vi "SP Format Marker Table.vi"(7 "CH Control In":T2={"Trace Orientation"=enum."Overlay", "Frequency"={"Change Frequency"=FALSE, "Start"=500.0, "Stop"=1500.0, "Units"=enum."MHz"}, "Markers"=[], "Traces"=[]} {"Traces"."Reference" format="%#.2g"; "Traces"."Display Data" items=["Data", "Memory", "Data/Memory"]; "Traces"."Format" items=["Log Mag", "Phase", "Expanded Phase", "Delay", "Smith", "Polar", "Lin Mag", "SWR", "Loss", "Real", "Imaginary"]; "Traces"."Scale" min=0.001 step=1.0 format="%#.2g"; "Traces"."Position" min=0.0 max=10.0; "Frequency"."Stop" format="%.3g"; "Frequency"."Start" format="%.3g"}, 8 "error in (no error)":errorcluster, 10 "Marker Table":refnum<vi>, 11 "Plot Ref":refnum<vi>) -> (0 "error out":errorcluster, 1 "Disable Button Values":T1)   [LabVIEW 2011]
uses:
  TypeDefs/SP Display Plot Controls Cluster.ctl
  TypeDefs/SP Frequency Units.ctl
  TypeDefs/SP Marker Cluster.ctl
  TypeDefs/SP Marker Type.ctl
  TypeDefs/SP Display Trace Controls.ctl
  TypeDefs/SP Display Format.ctl
  TypeDefs/SP Display Data.ctl
panel:
  # "Div"
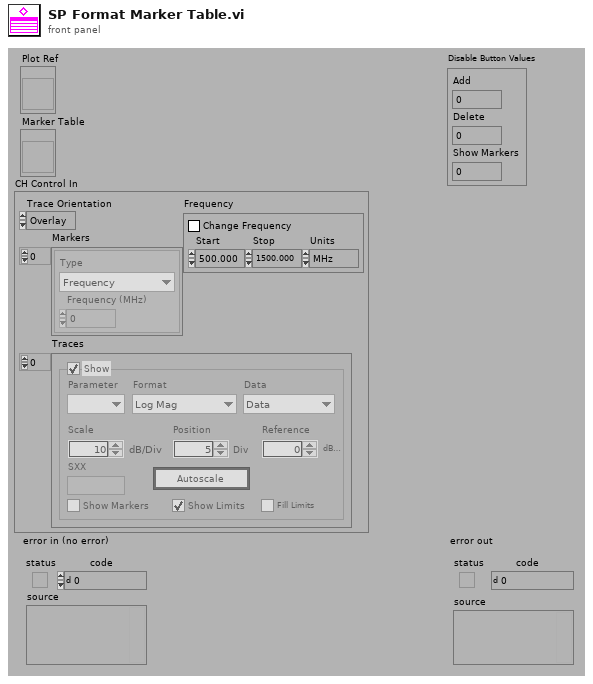
[diagram p1: front panel]
types:
  T1 = cluster{"Add":u8, "Delete":u8, "Show Markers":u8}
  T2 = typedef "SP Display Plot Controls Cluster.ctl" = cluster{"Trace Orientation":enum32{"Overlay", "Split"}, "Frequency":cluster{"Change Frequency":bool, "Start":dbl, "Stop":dbl, "Units":T3}, "Markers":T4[], "Traces":T6[]}
  T3 = typedef "SP Frequency Units.ctl" = enum16{"Hz", "kHz", "MHz", "GHz", "Points"}
  T4 = typedef "SP Marker Cluster.ctl" = cluster{"Type":T5, "Frequency (MHz)":dbl}
  T5 = typedef "SP Marker Type.ctl" = enum16{"Frequency", "Trace Maximum", "Trace Minimum", "Limit Maximum", "Limit Minimum"}
  T6 = typedef "SP Display Trace Controls.ctl" = cluster{"Trace On":bool, "Measure":i32, "Format":T7, "Autoscale":bool, "Reference":dbl, "\nRefUnit":string, "Position":dbl, "Scale":dbl, "ScaleUnit":string, "LimitOn":bool, "LimitFill":bool, "Display Data":T8, "Show Markers":bool, "SXX":string}
  T7 = typedef "SP Display Format.ctl" = i32
  T8 = typedef "SP Display Data.ctl" = u16
  T9 = typedef "SP Channel Data.ctl" = cluster{"Graph Ref":refnum<vi>, "Data":cluster{"Data":cluster{"X":dbl[], "Y":dbl[]}, "Index":i32}, "ULimits":cluster{"Data":cluster{"X":dbl[], "Y":dbl[]}, "Index":i32}[], "LLimits":cluster{"Data":cluster{"X":dbl[], "Y":dbl[]}, "Index":i32}[]}
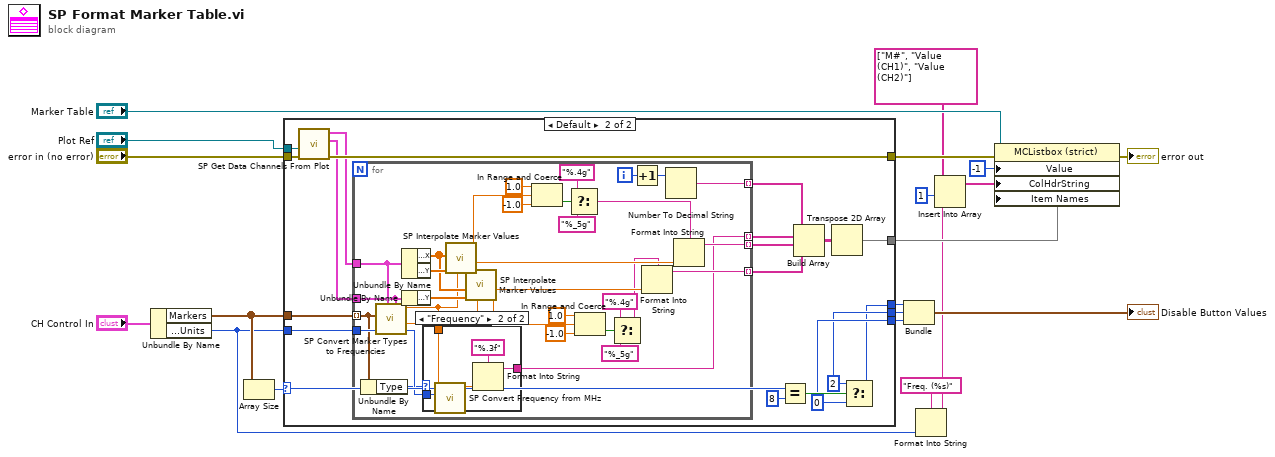
[diagram p0: block diagram]
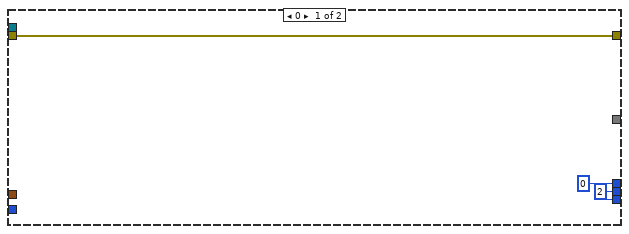
[diagram p2: hidden frame]
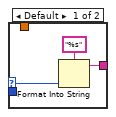
[diagram p3: hidden frame]
diagram:
  n1 = Unbundle By Name("CH Control In") -> ("Markers"=w2:T4[], "Frequency.Units"=w1:T3)
  n2 = Array Size(array=w2) -> (size(s)=w17:i32)
  n3 = case shown="Default" w17 {
    selector: w17 -> [_ w32]
    tunnel: w2 -> [_ w42]
    tunnel: "error in (no error)" -> [w23 w41]
    tunnel: [w23 w40] -> w11
    tunnel: "Plot Ref" -> [_ w39]
    tunnel: [_ w33] -> w12
    tunnel: [u8 0 w24] -> w15
    tunnel: [w22 w27] -> w14
    tunnel: [w22 w29] -> w13
    tunnel: w1 -> [_ w26]
    frame 0 {
      w22 = u8 2
    }
    frame Default {
      w29 = u8 0
      w27 = u8 2
      n4 = call "SP Get Data Channels From Plot.vi"("error in (no error)"=w41, "Plot Ref"=w39) -> ("error out"=w40:errorcluster, "CH 2"=w35:T9, "CH 1"=w36:T9)  [unwired: 7 out]
      n5 = for {
        tunnel: w42 -> [w45] mode=indexing
        tunnel: w35 -> [w47]
        tunnel: w36 -> [w48]
        tunnel: [w72] -> w37 mode=indexing
        tunnel: [w71] -> w38 mode=indexing
        tunnel: [w70] -> w25 mode=indexing
        tunnel: [w67] -> w28 mode=indexing
        tunnel: w26 -> [w66]
        i -> [w69]
        n6 = Unbundle By Name(w45) -> ("Type"=w44:T5)
        n7 = call "SP Convert Marker Types to Frequencies.vi"("CH 2"=w47, "CH 1"=w48, "Marker"=w45) -> ("CH2 Frequency"=w46:dbl, "CH1 Frequency"=w43:dbl)  [unwired: 5 out]
        n8 = Unbundle By Name(w48) -> ("Data.Data.X"=w63:dbl[], "Data.Data.Y"=w64:dbl[])
        n9 = Unbundle By Name(w47) -> ("Data.Data.Y"=w65:dbl[])
        n10 = case shown="\"Frequency\"" w44 {
          selector: w44 -> [w73 _]
          tunnel: [w74 w79] -> w70
          tunnel: w66 -> [_ w77]
          tunnel: w43 -> [_ w76]
          frame Default {
            n11 = Format Into String(format string="%s", w73) -> (resulting string=w74:string)  [unwired: 2 in, 1 out]
          }
          frame "Frequency" {
            n12 = call "SP Convert Frequency from MHz.vi"("Units"=w77, "Frequency (MHz)"=w76) -> ("Converted Frequency"=w78:dbl)  [unwired: 1 in, 8 out]
            n13 = Format Into String(format string="%.3f", w78) -> (resulting string=w79:string)  [unwired: 2 in, 1 out]
          }
        }
        n14 = call "SP Interpolate Marker Values.vi"("Marker Value"=w43, "Y Values"=w64, "X Values"=w63) -> ("Interpolated Y Value"=w57:dbl)  [unwired: 8 out]
        n15 = call "SP Interpolate Marker Values.vi"("Marker Value"=w46, "Y Values"=w65, "X Values"=w63) -> ("Interpolated Y Value"=w50:dbl)  [unwired: 8 out]
        n16 = In Range and Coerce(upper limit=1.0, x=w57, lower limit=-1.0) -> (In Range?=w59:bool)  [unwired: 1 out]
        n17 = Select(t="%.4g" ("format string"), s=w59, f="%_5g" ("format string")) -> (s? t:f=w56:string)
        n18 = In Range and Coerce(upper limit=1.0, x=w50, lower limit=-1.0) -> (In Range?=w54:bool)  [unwired: 1 out]
        n19 = Select(t="%.4g" ("format string"), s=w54, f="%_5g" ("format string")) -> (s? t:f=w49:string)
        n20 = Increment(x=w69) -> (x+1=w68:i32)
        n21 = Format Into String(format string=w49, w50) -> (resulting string=w72:string)  [unwired: 2 in, 1 out]
        n22 = Number To Decimal String(number=w68) -> (decimal integer string=w67:string)  [unwired: 1 out]
        n23 = Format Into String(format string=w56, w57) -> (resulting string=w71:string)  [unwired: 2 in, 1 out]
      }
      n24 = Equal?(x=w32, y=8) -> (x = y?=w30:bool)
      n25 = Build Array(w28, w25, w38, w37) -> (w34:string[][])
      n26 = Transpose 2D Array(2D array=w34) -> (transposed array=w33:string[][])
      n27 = Select(t=w27, s=w30, f=w29) -> (s? t:f=w24:u8)
    }
  }
  n28 = Bundle(w15, w14, w13) -> (→"Disable Button Values":cluster{u8, u8, u8})  [unwired: 1 out]
  n29 = Format Into String(format string="Freq. (%s)", w1) -> (resulting string=w5:string)  [unwired: 2 in, 1 out]
  n30 = Insert Into Array(array=string[] ["M#", "Value (CH1)", "Value (CH2)"] ("t"), index=1, new element=w5) -> (w6:string[])
  n31 = property class="MCListbox (strict)"(reference="Marker Table", error in=w11, "Value"=-1 ("Value (Signaling)"), "ColHdrString"=w6, "Item Names"=w12) -> (error out=→"error out":errorcluster)  [unwired: 1 out]
